vi "Set message.vi"(10 "WampMessage MsgPack":refnum<class "WampMessage MsgPack.lvclass">, 11 "HandleSubscribed MsgPack in":refnum<class "HandleSubscribed MsgPack.lvclass">) -> (3 "HandleSubscribed MsgPack out":refnum<class "HandleSubscribed MsgPack.lvclass">)   [LabVIEW 2020, in "wamplv.lvlib" / "HandleSubscribed MsgPack.lvclass"]
uses:
  HandleSubscribed MsgPack.lvclass
  HandleSubscribed MsgPack.lvclass/HandleSubscribed MsgPack.ctl
  SerialisedMessages/MsgPackMessage/WampMessage MsgPack.lvclass
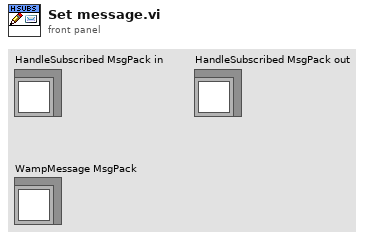
[diagram p1: front panel]
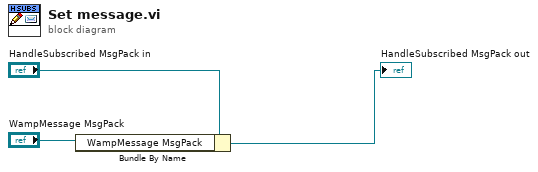
[diagram p0: block diagram]
diagram:
  n1 = Bundle By Name(cluster="HandleSubscribed MsgPack in", "WampMessage MsgPack"="WampMessage MsgPack") -> (→"HandleSubscribed MsgPack out":refnum<class "HandleSubscribed MsgPack.lvclass">)
